vi "Payload to String.vi"(3 "Payload":string) -> (1 "String":string)   [LabVIEW 2019]
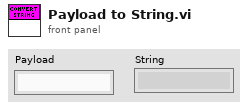
[diagram p1: front panel]
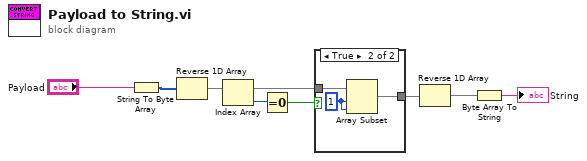
[diagram p0: block diagram]
diagram:
  n1 = String To Byte Array(string="Payload") -> (unsigned byte array=w8:u8[])
  n2 = Reverse 1D Array(array=w8) -> (reversed array=w5:u8[])
  n3 = Index Array(array=w5) -> (element=w7:u8)  [unwired: 1 in]
  n4 = Equal To 0?(x=w7) -> (x = 0?=w6:bool)
  n5 = case shown="True" w6 {
    tunnel: w5 -> [w9 w12]
    tunnel: [w9 w11] -> w4
    frame False {
    }
    frame True {
      w10 = 1 ("index")
      n6 = Array Subset(array=w12, index=w10, length=w10) -> (w11:u8[])
    }
  }
  n7 = Reverse 1D Array(array=w4) -> (reversed array=w3:u8[])
  n8 = Byte Array To String(unsigned byte array=w3) -> (string=→"String":string)
